vi "Holding Var.vi"() -> ()   [LabVIEW 2016, in "EXO2-Sonde.lvlib"]
uses:
  EXO2-Sonde.lvlib
panel:
  in  "测试间隔":u16=1
  in  "baud rate (9600)":u32=38400
  in  "EXO串口":refnum<visa-resource-name>="COM4"
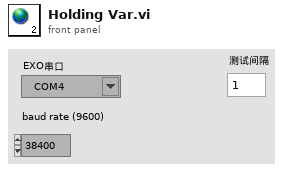
[diagram p1: front panel]
diagram:
